vi "DeferPanelUpdates.vi"(8 "error in (no error)":errorcluster, 10 "Defer Panel Updates":bool, 11 "VI in":refnum<vi>) -> (0 "error out":errorcluster)   [LabVIEW 2023]
panel:
  # "Output"
  # "Input"
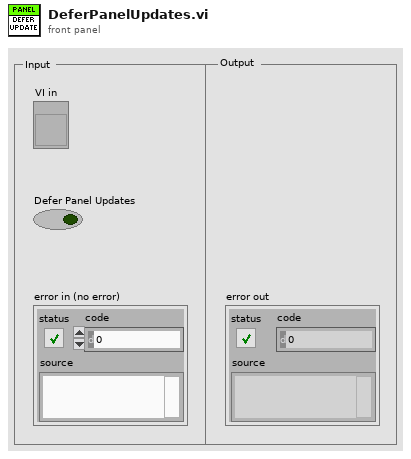
[diagram p1: front panel]
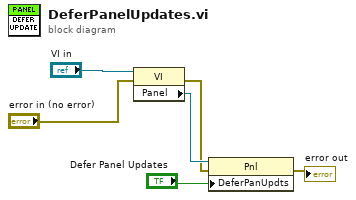
[diagram p0: block diagram]
diagram:
  n1 = property class="VI"(reference="VI in", error in="error in (no error)") -> (error out=w1:errorcluster, "Panel"=w5:refnum<vi>)  [unwired: 1 out]
  n2 = property class="Pnl"(reference=w5, error in=w1, "DeferPanUpdts"="Defer Panel Updates") -> (error out=→"error out":errorcluster)  [unwired: 1 out]
